vi "Yokogawa Control.vi"(8 "error in (no error)":errorcluster, 10 "Master":refnum<queue>, 11 "reference":refnum<vi>) -> (0 "error out":errorcluster)   [LabVIEW 2014, in "Instrument Launcher.lvlib"]
uses:
  Support/MeasurementControl Message Queue Folder/Message Cluster.ctl
  Instrument Launcher.lvlib
  Support/MeasurementControl Message Queue Folder/MeasurementControl Message Queue.lvlib
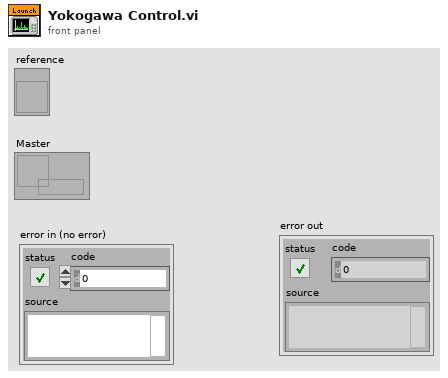
[diagram p1: front panel]
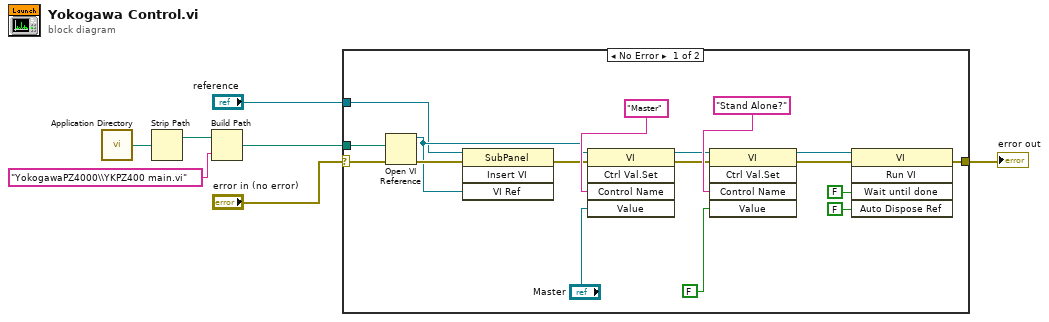
[diagram p0: block diagram]
diagram:
  n1 = call <vilib>:"Application Directory.vi"() -> ("Application Directory"=w2:path)
  n2 = Strip Path(path=w2) -> (stripped path=w3:path)  [unwired: 1 out]
  n3 = Build Path(base path=w3, name or relative path="YokogawaPZ4000\\YKPZ400 main.vi") -> (appended path=w1:path)
  n4 = case shown="No Error" "error in (no error)" {
    selector: "error in (no error)" -> [w8 w25]
    tunnel: w1 -> [w15 _]
    tunnel: "reference" -> [w13 _]
    tunnel: [w11 w25] -> w6
    frame No Error {
      n5 = Open VI Reference(vi path=w15, error in (no error)=w8) -> (vi reference=w14:refnum<vi>, error out=w16:errorcluster)  [unwired: 4 in]
      n6 = invoke on="Invoke Node" class="SubPanel" method="Insert VI"(reference=w13, error in=w16, "VI Ref"=w14) -> (error out=w12:errorcluster)  [unwired: 1 in, 3 out]
      n7 = invoke class="VI" method="Ctrl Val.Set"(reference=w14, error in=w12, "Control Name"="Master", "Value"="Master") -> (reference out=w10:refnum<vi>, error out=w9:errorcluster)  [unwired: 1 in, 3 out]
      n8 = invoke class="VI" method="Ctrl Val.Set"(reference=w10, error in=w9, "Control Name"="Stand Alone?", "Value"=FALSE) -> (reference out=w19:refnum<vi>, error out=w18:errorcluster)  [unwired: 1 in, 3 out]
      n9 = invoke class="VI" method="Run VI"(reference=w19, error in=w18, "Wait until done"=FALSE ("Wait Until Done"), "Auto Dispose Ref"=FALSE ("Auto Dispose Reference")) -> (error out=w11:errorcluster)  [unwired: 1 in, 4 out]
    }
    frame Error {
    }
  }
  "error out" <- w6
